vi "xyTest.vi"() -> ()   [LabVIEW 2012]
panel:
  out "XY Graph":cluster{"Array":dbl[], "Array 3":dbl[]}[](graph)=[{"Array"=[1.0, 2.0, 3.0, 4.0, 5.0, 6.0], "Array 3"=[1.0, 4.0, 9.0, 16.0, 25.0, 36.0]}, {"Array"=[1.0, 2.0, 3.0, 4.0, 5.0, 6.0], "Array 3"=[10.0, 8.0, 6.0, 4.0, 2.0, 0.0]}]
  in  "Array 3":dbl[](array[numeric])=[10.0, 8.0, 6.0, 4.0, 2.0, 0.0]
  in  "Array 2":dbl[](array[numeric])=[1.0, 4.0, 9.0, 16.0, 25.0, 36.0]
  in  "Array":dbl[](array[numeric])=[1.0, 2.0, 3.0, 4.0, 5.0, 6.0]
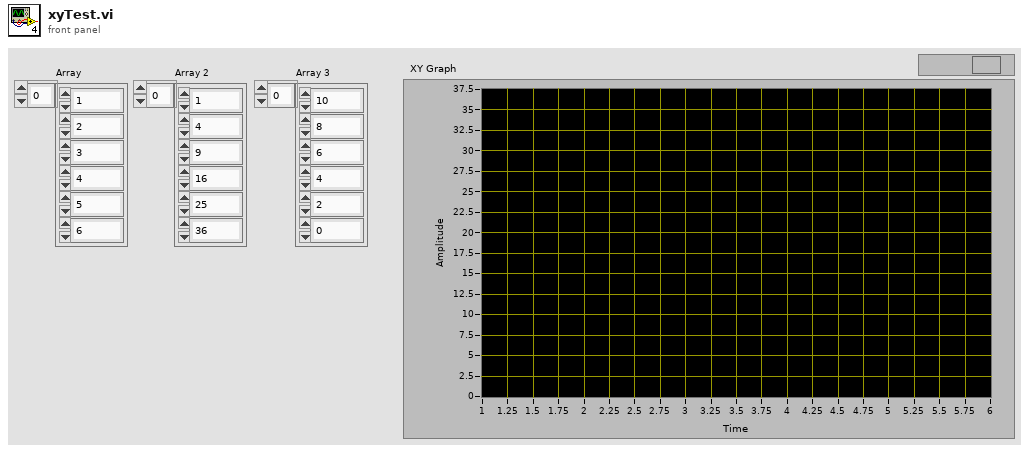
[diagram p1: front panel]
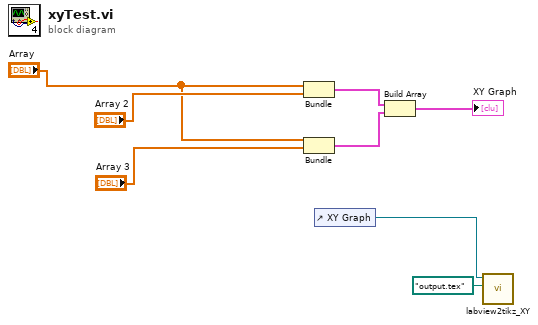
[diagram p0: block diagram]
diagram:
  n1 = Bundle("Array"="Array", "Array 2"="Array 2") -> (w5:cluster{"Array":dbl[], "Array 2":dbl[]})  [unwired: 1 in]
  n2 = Bundle("Array"="Array", "Array 3"="Array 3") -> (w4:cluster{"Array":dbl[], "Array 3":dbl[]})  [unwired: 1 in]
  n3 = control-ref of="XY Graph"() -> (w2:refnum<vi>)
  n4 = Build Array(w5, w4) -> (→"XY Graph":cluster{"Array":dbl[], "Array 3":dbl[]}[])
  n5 = call "labview2tikz_XY.vi"("file (use dialog)"=path "output.tex", "XY Graph 2"=w2) -> ()  [unwired: 8 in, 2 out]
